vi "1D Polar To Rectangular.vi"(1 "Magnitude":dbl[](array[numeric]) format="%0.2f", 4 "Phase":dbl[](array[numeric]) format="%0.2f") -> (0 "X":dbl[](array[numeric]) format="%0.2f", 2 "Y":dbl[](array[numeric]) format="%0.2f", 3 "error":i32)   [LabVIEW 2017, in "NI_AALPro.lvlib"]
doc: "LabVIEW no longer supports this VI. Use the Polar To Re/Im function instead.\nThis VI converts two arrays of polar coordinates represented by the input arrays <b>Magnitude</b> and <b>Phase</b> into two arrays of rectangular coordinates.\nThis VI converts the arrays of polar coordinates into arrays of rectangular coordinates using the following equations.\n<b>X</b> = <b>Magnitude</b>*cos(<b>Phase</b>)\n<b>Y</b> = <b>Magnitude</b>*sin(<b>Phase</b>)"
uses:
  NI_AALPro.lvlib
  lvanlys.dll
panel:
  # "1D Polar To Rectangular"
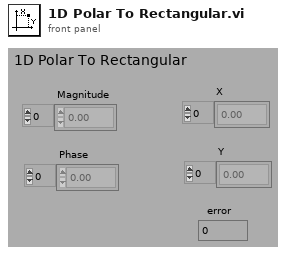
[diagram p1: front panel]
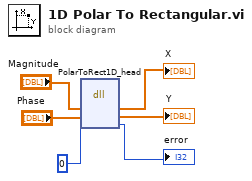
[diagram p0: block diagram]
diagram:
  n1 = dll-call lib="C:/Program Files/National Instruments/LabVIEW 2017/resource/lvanlys.*" fn="PolarToRect1D_head"("Magnitude"="Magnitude", "Phase"="Phase", 0) -> ("Magnitude"=→"X":dbl[], "Phase"=→"Y":dbl[], →"error":i32)  [unwired: 4 in, 2 out]
